vi "(Incomplete) Beta Function.vi"   [LabVIEW 2020, in "NI_Gmath.lvlib"]
doc: "Evaluates the beta function and regularized incomplete beta function. You must manually select the polymorphic instance you want to use."
uses:
  <vilib>/gmath/NI_Gmath.lvlib
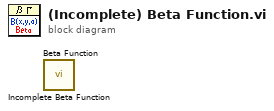
[diagram p0: block diagram]
diagram:
  n1 = call <vilib>:"Incomplete Beta Function.vi"() -> ()  [unwired: 11 in, 1 out]
  n2 = call <vilib>:"Beta Function.vi"() -> ()  [unwired: 11 in, 1 out]
